vi "Get Trigger Mode.vi"(8 "error in (no error)":errorcluster, 11 "FW102C in":i32) -> (0 "error out":errorcluster, 2 "Trigger Mode":enum16{"Input Mode", "Output Mode"}(ring), 3 "FW102C out":i32)   [LabVIEW 2018, in "Thorlabs_FW102C.lvlib"]
doc: "Returns the trigger mode"
uses:
  Thorlabs_FW102C.lvlib
  <instrlib>/Thorlabs_FW102C/Library/FilterWheel102_win32.dll
  Library/FilterWheel102_win64.dll
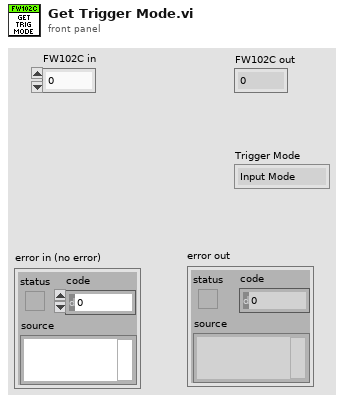
[diagram p1: front panel]
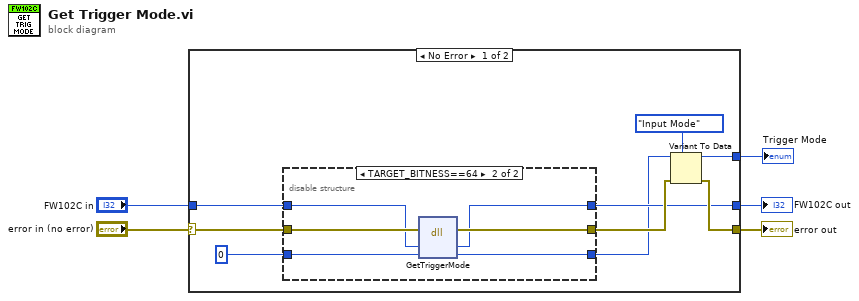
[diagram p0: block diagram]
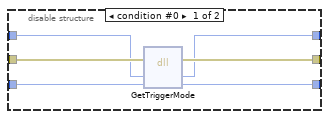
[diagram p2: hidden frame]
diagram:
  n1 = case shown="No Error" "error in (no error)" {
    selector: "error in (no error)" -> [w11 w27]
    tunnel: [w12 w27] -> w5
    tunnel: "FW102C in" -> [w9 w28]
    tunnel: [w8 w28] -> w2
    tunnel: [w14 _] -> w1
    frame No Error {
      n2 = disable-structure shown="TARGET_BITNESS==64" {
        disable-tunnel: w11 -> [w20 w26]
        disable-tunnel: [w19 w25] -> w10
        disable-tunnel: w9 -> [w18 w24]
        disable-tunnel: [w17 w23] -> w8
        disable-tunnel: [w16 w22] -> w7
        disable-tunnel: 0 ("trigger mode") -> [w15 w21]
        frame condition #0 {
          n3 = dll-call lib="E:/Program Files (x86)/National Instruments/LabVIEW 2011/instr.lib/Thorlabs_FW102C/Library/FilterWheel102_win32.dll" fn="GetTriggerMode"(error in=w20, "hdl"=w18, "trigger mode"=w15) -> (error out=w19:errorcluster, "hdl"=w17:i32, "trigger mode"=w16:i32)  [unwired: 3 in, 1 out]
        }
        frame condition #1 (active) {
          n4 = dll-call lib="C:/Users/astrolab/Desktop/Labview_code/Thorlabs_FW102C/Library/FilterWheel102_win64.dll" fn="GetTriggerMode"(error in=w26, "hdl"=w24, "trigger mode"=w21) -> (error out=w25:errorcluster, "hdl"=w23:i32, "trigger mode"=w22:i32)  [unwired: 3 in, 1 out]
        }
      }
      n5 = Variant To Data(error in=w10, type=enum16{"Input Mode", "Output Mode"}."Input Mode" ("Trigger Mode"), Variant=w7) -> (data=w14:enum16{"Input Mode", "Output Mode"}, error out=w12:errorcluster)
    }
    frame Error {
    }
  }
  "error out" <- w5
  "FW102C out" <- w2
  "Trigger Mode" <- w1
